vi "Rec Fetch Recordset Data (R).vi"(4 "error in (no error)":errorcluster, 7 "recordset reference":T1) -> (0 "error out":errorcluster, 1 "recordset data":variant[][](array[variant]), 3 "recordset reference out":T1)   [LabVIEW 2017, in "NI_Database_API.lvlib"]
doc: "Retrieves the data in the recordset identified by the <B>recordset reference</B> input. You can convert each element in the array to its native LabVIEW data type using the Database Variant To Data function. Wire data to the reference input to determine the polymorphic instance to use or manually select the instance."
uses:
  <vilib>/addons/database/NI_Database_API.lvlib
  <vilib>/addons/database/Recordset.llb/Rec ObjectReference.ctl
  <vilib>/addons/database/Recordset.llb/Rec Get Recordset Properties (R).vi
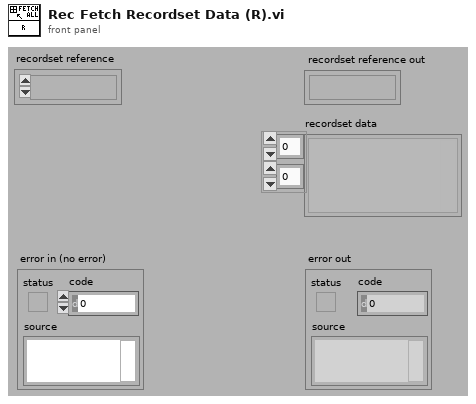
[diagram p1: front panel]
types:
  T1 = typedef "NI_Database_API.lvlib/Rec ObjectReference.ctl" = refnum<k1>
  T2 = typedef "NI_Database_API.lvlib/Rec Properties.ctl" = cluster{"column count":i32, "record index":i32, "record count":i32, "bof?":bool, "eof?":bool, "cursor type":T3, "cache size":i32, "state":enum16{"closed", "open"}}
  T3 = typedef "NI_Database_API.lvlib/DB Tools Cursor Type.ctl" = enum16{"forward-only", "keyset", "dynamic", "static"}
  T4 = typedef "NI_Database_API.lvlib/Rec DataMembers.ctl" = cluster{"ADODB._Recordset":refnum<k7>, "Connection":T5}
  T5 = typedef "NI_Database_API.lvlib/Conn ObjectReference.ctl" = refnum<k1>
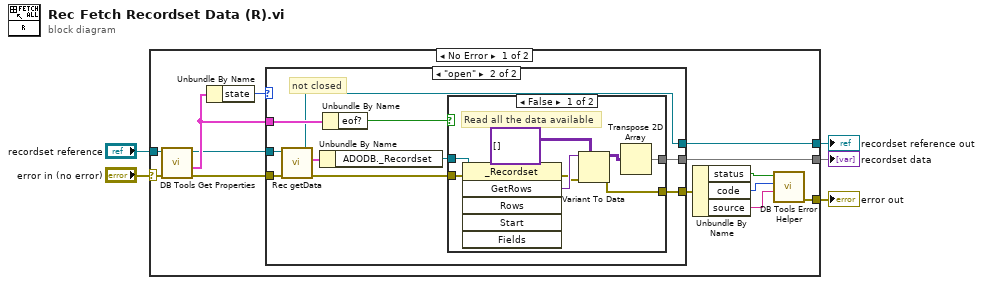
[diagram p0: block diagram]
diagram:
  n1 = case shown="No Error" "error in (no error)" {
    selector: "error in (no error)" -> [w13 w41]
    tunnel: [w7 w41] -> w5
    tunnel: "recordset reference" -> [w14 w40]
    tunnel: [w12 w40] -> w3
    tunnel: [w6 _] -> w2
    frame No Error {
      n2 = call-poly <vilib>:"DB Tools Get Properties.vi"("error in (no error)"=w13, "recordset reference"=w14) -> ("error out"=w16:errorcluster, "recordset properties"=w18:T2, "recordset reference out"=w15:T1)  [unwired: 3 out]
      n3 = Unbundle By Name(w18) -> ("state"=w17:enum16{"closed", "open"})
      n4 = case shown="\"open\"" w17 {
        tunnel: w16 -> [w19 w25]
        tunnel: [w20 w22] -> w12
        tunnel: [w19 w30] -> w8
        tunnel: [_ w29] -> w6
        tunnel: w15 -> [w20 w26]
        tunnel: w18 -> [_ w28]
        frame "closed" {
          # "The object is closed so pass out an empty 2-D array"
        }
        frame "open" {
          # "not closed"
          n5 = call <vilib>:"Rec getData.vi"("error in (no error)"=w25, "recordset reference"=w26) -> ("error out"=w24:errorcluster, "data"=w27:T4, "recordset reference out"=w22:T1)  [unwired: 3 out]
          n6 = Unbundle By Name(w27) -> ("ADODB._Recordset"=w23:refnum<k7>)
          n7 = Unbundle By Name(w28) -> ("eof?"=w21:bool)
          n8 = case shown="False" w21 {
            tunnel: w24 -> [w35 w39]
            tunnel: [w34 w39] -> w30
            tunnel: [w33 _] -> w29
            tunnel: w23 -> [w32 _]
            frame False {
              # "Read all the data available"
              n9 = invoke class="_Recordset" method="GetRows"(reference=w32, error in=w35) -> (error out=w36:errorcluster, "GetRows"=w37:variant)  [unwired: 4 in, 4 out]
              n10 = Variant To Data(error in=w36, type=variant[][] [], Variant=w37) -> (data=w38:variant[][], error out=w34:errorcluster)
              n11 = Transpose 2D Array(2D array=w38) -> (transposed array=w33:variant[][])
            }
            frame True {
              # "If (beginning of file and end of file) or  end of file are true, then the recordset is empty and there is nothing to fetch."
            }
          }
        }
      }
      n12 = Unbundle By Name(w8) -> ("status"=w10:bool, "code"=w11:i32, "source"=w9:string)
      n13 = call <vilib>:"DB Tools Error Helper.vi"("source"=w9, "code"=w11, "status"=w10) -> ("error out"=w7:errorcluster)  [unwired: 1 in, 7 out]
    }
    frame Error {
    }
  }
  "recordset reference out" <- w3
  "error out" <- w5
  "recordset data" <- w2
